vi "oa_Get Actual Max Order.vi"(9 "max order (auto)":dbl, 10 "pulse/revolution (1)":i32=1, 11 "max suggested order":dbl) -> (1 "new pulse/revolution":dbl, 3 "interpolation factor":i32)   [LabVIEW 2017, in "SoundVib_Resampling.lvlib"]
uses:
  <vilib>/addons/Sound and Vibration/Order Analysis/Resample Order Tracking/SoundVib_Resampling.lvlib
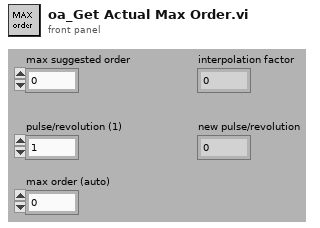
[diagram p1: front panel]
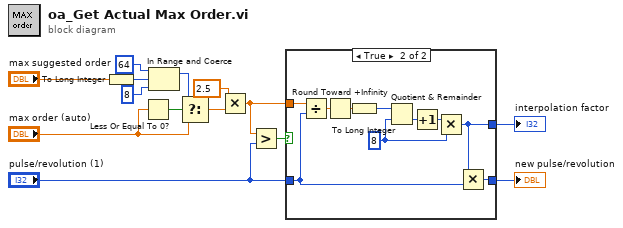
[diagram p0: block diagram]
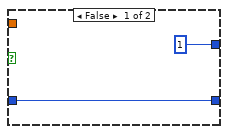
[diagram p2: hidden frame]
diagram:
  n1 = To Long Integer(number="max suggested order") -> (32bit integer=w12:i32)
  n2 = Less Or Equal To 0?(x="max order (auto)") -> (x <= 0?=w6:bool)
  n3 = In Range and Coerce(upper limit=64 ("x"), x=w12, lower limit=8) -> (coerced(x)=w14:i32)  [unwired: 1 out]
  n4 = Select(t=w14, s=w6, f="max order (auto)") -> (s? t:f=w10:dbl)
  n5 = Multiply(x=2.5, y=w10) -> (x*y=w4:dbl)
  n6 = Greater?(x=w4, y="pulse/revolution (1)") -> (0:w5:bool)
  n7 = case shown="True" w5 {
    tunnel: w4 -> [_ w26]
    tunnel: "pulse/revolution (1)" -> [w15 w17]
    tunnel: [1 w18] -> w2
    tunnel: [w15 w19] -> w1
    frame False {
    }
    frame True {
      w25 = 8 ("y")
      n8 = Divide(x=w26, y=w17) -> (x/y=w22:dbl)
      n9 = Round Toward +Infinity(x=w22) -> (ceil(x): smallest int >= x=w21:dbl)
      n10 = To Long Integer(number=w21) -> (32bit integer=w20:i32)
      n11 = Quotient & Remainder(x=w20, y=w25) -> (floor(x/y)=w23:i32)  [unwired: 1 out]
      n12 = Increment(x=w23) -> (x+1=w24:i32)
      n13 = Multiply(x=w24, y=w25) -> (x*y=w18:i32)
      n14 = Multiply(x=w18, y=w17) -> (x*y=w19:i32)
    }
  }
  "interpolation factor" <- w2
  "new pulse/revolution" <- w1
